vi "GetDeleteChannel.vi"(7 "CHANNEL":string[][](array[string]), 10 "CtlRef":refnum<vi>) -> (1 "Finded":bool, 2 "通道":string[](array[string]))   [LabVIEW 2015]
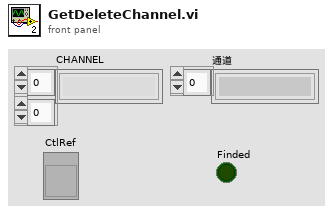
[diagram p1: front panel]
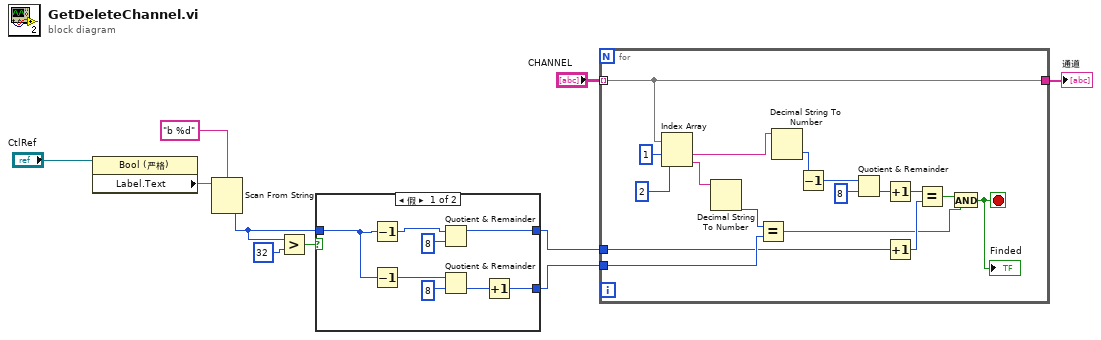
[diagram p0: block diagram]
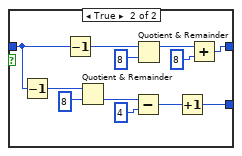
[diagram p2: hidden frame]
diagram:
  n1 = property class="Bool (严格)"(reference="CtlRef") -> ("Label.Text"=w8:string)  [unwired: 1 in, 2 out]
  n2 = Scan From String(format string="b %d", input string=w8) -> (output 1=w7:i32)  [unwired: 3 in, 3 out]
  n3 = Greater?(x=w7, y=32) -> (0:w5:bool)
  n4 = case shown="假" w5 {
    tunnel: [w15 w19] -> w1
    tunnel: [w11 w26] -> w3
    tunnel: w7 -> [w13 w23]
    frame False {
      n5 = Decrement(x=w13) -> (x-1=w12:i32)
      n6 = Decrement(x=w13) -> (x-1=w18:i32)
      n7 = Quotient & Remainder(x=w12, y=8) -> (x-y*floor(x/y)=w11:i32)  [unwired: 1 out]
      n8 = Quotient & Remainder(x=w18, y=8) -> (floor(x/y)=w16:i32)  [unwired: 1 out]
      n9 = Increment(x=w16) -> (x+1=w15:i32)
    }
    frame True {
      n10 = Decrement(x=w23) -> (x-1=w25:i32)
      n11 = Decrement(x=w23) -> (x-1=w30:i32)
      n12 = Quotient & Remainder(x=w25, y=8) -> (floor(x/y)=w22:i32)  [unwired: 1 out]
      n13 = Subtract(x=w22, y=4) -> (x-y=w20:i32)
      n14 = Quotient & Remainder(x=w30, y=8) -> (x-y*floor(x/y)=w28:i32)  [unwired: 1 out]
      n15 = Increment(x=w20) -> (x+1=w19:i32)
      n16 = Add(x=w28, y=8) -> (x+y=w26:i32)
    }
  }
  n17 = for {
    tunnel: "CHANNEL" -> [w47] mode=indexing
    tunnel: [w47] -> w2
    tunnel: w1 -> [w46]
    tunnel: w3 -> [w42]
    stop <- w37 stop-if-true
    n18 = Index Array(array=w47, index #1=1 ("index"), index #2=2 ("index")) -> (element #1=w34:string, element #2=w32:string)
    n19 = Decimal String To Number(string=w32) -> (number=w31:i32)  [unwired: 2 in, 1 out]
    n20 = Equal?(x=w31, y=w46) -> (x = y?=w38:bool)
    n21 = Decimal String To Number(string=w34) -> (number=w33:i32)  [unwired: 2 in, 1 out]
    n22 = Decrement(x=w33) -> (x-1=w45:i32)
    n23 = Quotient & Remainder(x=w45, y=8) -> (floor(x/y)=w43:i32)  [unwired: 1 out]
    n24 = Increment(x=w43) -> (x+1=w41:i32)
    n25 = Increment(x=w42) -> (x+1=w40:i32)
    n26 = Equal?(x=w41, y=w40) -> (x = y?=w39:bool)
    n27 = And(x=w39, y=w38) -> (x .and. y?=w37:bool)
    "Finded" <- w37
  }
  "通道" <- w2
